vi "Obliczanie_symptomów (SubVI).vi"(0 "V [obr/min]":dbl, 3 "fs [Hz]":dbl) -> (7 "Prêdkoœæ synchroniczna":dbl, 8 "Poœlizg":dbl, 9 "fp +":dbl, 10 "fp -":dbl)   [LabVIEW 2018]
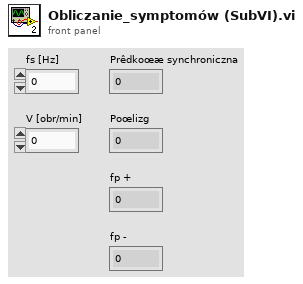
[diagram p1: front panel]
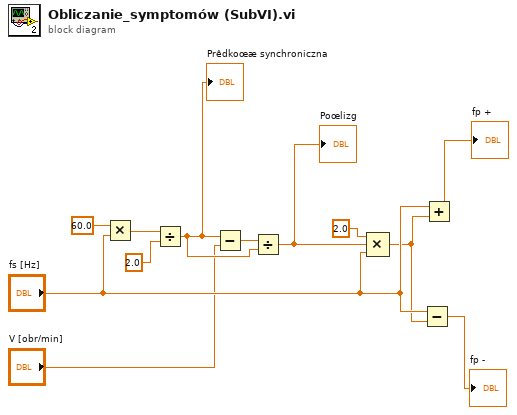
[diagram p0: block diagram]
diagram:
  n1 = Multiply(x=60.0, y="fs [Hz]") -> (x*y=w2:dbl)
  n2 = Divide(x=w2, y=2.0) -> (x/y=w6:dbl)
  "Prêdkoœæ synchroniczna" <- w6
  n3 = Subtract(x=w6, y="V [obr/min]") -> (x-y=w4:dbl)
  n4 = Divide(x=w4, y=w6) -> (x/y=w9:dbl)
  "Poœlizg" <- w9
  n5 = Compound Arithmetic op=MULTIPLY(2.0 ("value"), w9, "fs [Hz]") -> (w7:dbl)
  n6 = Subtract(x="fs [Hz]", y=w7) -> (x-y=→"fp -":dbl)
  n7 = Add(x="fs [Hz]", y=w7) -> (x+y=→"fp +":dbl)
